vi "logic_block.vi"(2 "Control":T3, 3 "B":T4, 4 "A":T5) -> (0 "Flags":T1, 1 "Result":T2)   [LabVIEW 2013]
panel:
  # "R1"
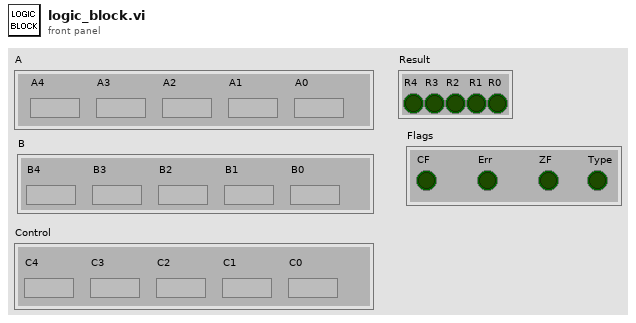
[diagram p1: front panel]
types:
  T1 = cluster{"CF":bool, "Err":bool, "ZF":bool, "Type":bool}
  T2 = cluster{"R4":bool, "R3":bool, "R2":bool, bool, "R0":bool}
  T3 = cluster{"C4":bool, "C3":bool, "C2":bool, "C1":bool, "C0":bool}
  T4 = cluster{"B4":bool, "B3":bool, "B2":bool, "B1":bool, "B0":bool}
  T5 = cluster{"A4":bool, "A3":bool, "A2":bool, "A1":bool, "A0":bool}
  T6 = cluster{"Result":cluster{"R4":bool, "R3":bool, "R2":bool, bool, "R0":bool}, "Result":cluster{"R4":bool, "R3":bool, "R2":bool, bool, "R0":bool}, "Result":cluster{"R4":bool, "R3":bool, "R2":bool, bool, "R0":bool}, "Result":cluster{"R4":bool, "R3":bool, "R2":bool, bool, "R0":bool}}
  T7 = cluster{"Flags":cluster{"CF":bool, "Err":bool, "ZF":bool, "Type":bool}, "Flags":cluster{"CF":bool, "Err":bool, "ZF":bool, "Type":bool}, "Flags":cluster{"CF":bool, "Err":bool, "ZF":bool, "Type":bool}, "Flags":cluster{"CF":bool, "Err":bool, "ZF":bool, "Type":bool}}
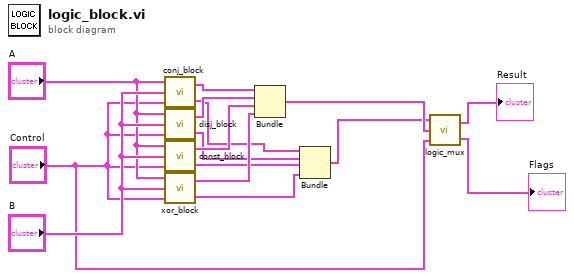
[diagram p0: block diagram]
diagram:
  n1 = call "conj_block.vi"("Control"="Control", "B"="B", "A"="A") -> ("Flags"=w9:T1, "Result"=w13:T2)
  n2 = call "disj_block.vi"("Control"="Control", "B"="B", "A"="A") -> ("Flags"=w8:T1, "Result"=w12:T2)
  n3 = call "const_block.vi"("Control"="Control", "B"="B", "A"="A") -> ("Flags"=w7:T1, "Result"=w11:T2)
  n4 = call "xor_block.vi"("Control"="Control", "B"="B", "A"="A") -> ("Flags"=w6:T1, "Result"=w10:T2)
  n5 = Bundle("Result"=w13, "Result"=w12, "Result"=w11, "Result"=w10) -> (w5:T6)  [unwired: 1 in]
  n6 = Bundle("Flags"=w9, "Flags"=w8, "Flags"=w7, "Flags"=w6) -> (w1:T7)  [unwired: 1 in]
  n7 = call "logic_mux.vi"("Control"="Control", "Input_results"=w5, "Input_flags"=w1) -> ("Flags"=→"Flags":T1, "Result"=→"Result":T2)
